vi "fg_width_padding.vi"(8 "error in (no error)":errorcluster) -> (0 "error out":errorcluster, 3 "width_padding":u32=10)   [LabVIEW 2015, in "lv-pagination.lvlib"]
uses:
  lv-pagination.lvlib
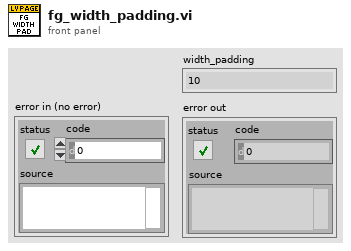
[diagram p1: front panel]
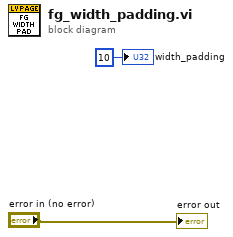
[diagram p0: block diagram]
diagram:
  "error out" <- "error in (no error)"
  "width_padding" <- u32 10 ("x")
